vi "TCP-Send Command Receive Double.vi"(0 "PXI Address":string, 5 "Port":i32, 7 "Command":string, 9 "timeout (ms)":i32=5000, 11 "error in (no error)":errorcluster) -> (4 "value":dbl, 10 "result":i32, 15 "error out":errorcluster)   [LabVIEW 2020]
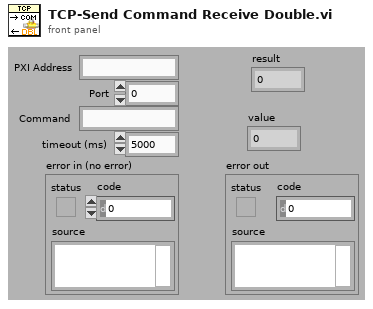
[diagram p1: front panel]
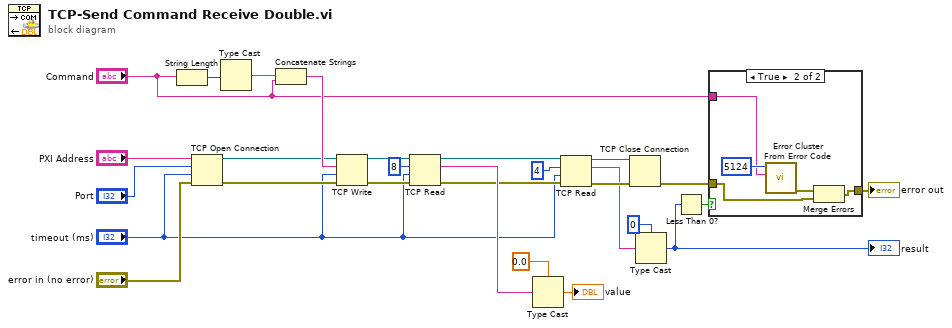
[diagram p0: block diagram]
diagram:
  n1 = String Length(string="Command") -> (length=w23:i32)
  n2 = TCP Open Connection(address="PXI Address", remote port or service name="Port", timeout ms (60000)="timeout (ms)", error in (no error)="error in (no error)") -> (connection ID=w20:refnum<k5>, error out=w21:errorcluster)  [unwired: 1 in]
  n3 = Type Cast(x=w23) -> (*(type *) &x=w22:string)  [unwired: 1 in]
  n4 = Concatenate Strings(w22, "Command") -> (w24:string)
  n5 = TCP Write(connection ID=w20, data in=w24, error in (no error)=w21, 9:"timeout (ms)") -> (connection ID out=w9:refnum<k5>, error out=w8:errorcluster)  [unwired: 1 out]
  n6 = TCP Read(connection ID=w9, bytes to read=8, error in (no error)=w8, 9:"timeout (ms)") -> (connection ID out=w7:refnum<k5>, data out=w6:string, error out=w5:errorcluster)  [unwired: 1 in]
  n7 = Type Cast(type=0.0, x=w6) -> (*(type *) &x=→"value":dbl)
  n8 = TCP Read(connection ID=w7, bytes to read=4, error in (no error)=w5, 9:"timeout (ms)") -> (connection ID out=w17:refnum<k5>, data out=w16:string, error out=w18:errorcluster)  [unwired: 1 in]
  n9 = TCP Close Connection(connection ID=w17, error in (no error)=w18) -> (error out=w11:errorcluster)  [unwired: 1 in, 1 out]
  n10 = Type Cast(type=0, x=w16) -> (*(type *) &x=w14:i32)
  "result" <- w14
  n11 = Less Than 0?(x=w14) -> (x < 0?=w13:bool)
  n12 = case shown="True" w13 {
    tunnel: [w28 w30] -> w12
    tunnel: w11 -> [w28 w29]
    tunnel: "Command" -> [_ w31]
    frame False {
    }
    frame True {
      n13 = call <vilib>:"Error Cluster From Error Code.vi"("error message (\"\")"=w31, "error code (0)"=5124) -> ("error out"=w33:errorcluster)  [unwired: 7 in]
      n14 = Merge Errors(w33, w29) -> (w30:errorcluster)
    }
  }
  "error out" <- w12
